vi "删除无效的文件路径.vi"(8 "error in (no error)":errorcluster, 10 "Enum":enum16{".xls", ".txt"}(ring), 11 "NewVal":string[](array[string])) -> (0 "error out":errorcluster, 2 "FilePathArray":path[](array[path]), 3 "NewVal 2":string[](array[string]))   [LabVIEW 2012]
doc: "从树形结构中选择的多个文件，有些是无效的文件路径（文件夹路径），需要删除。\n\nName:蒋松\nEmail:jiangsong@outlook.com"
panel:
  # "VI INPUTS"
  # "VI OUTPUTS"
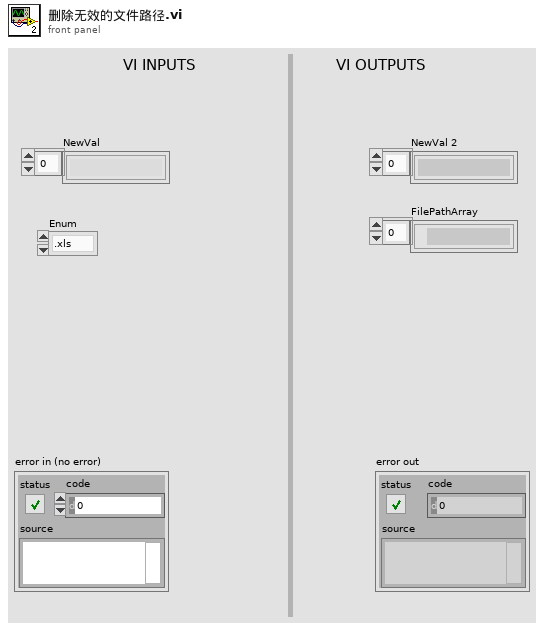
[diagram p1: front panel]
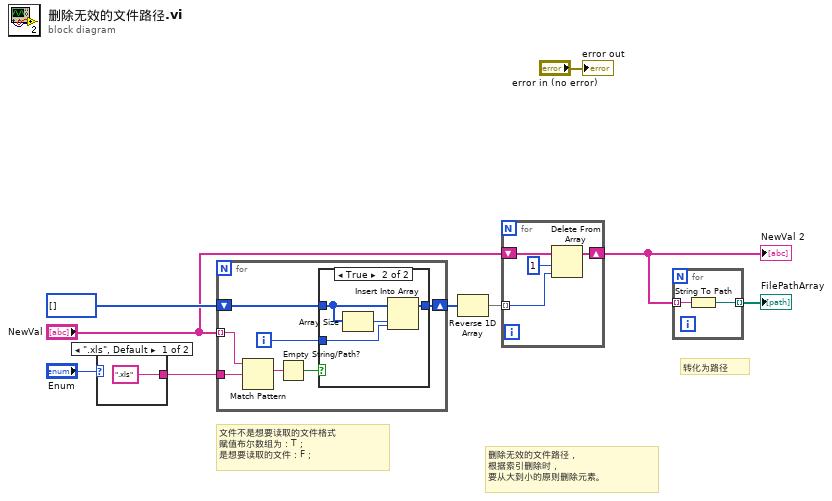
[diagram p0: block diagram]
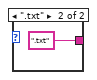
[diagram p2: hidden frame]
diagram:
  # "转化为路径"
  # "删除无效的文件路径，\n根据索引删除时，\n要从大到小的原则删除元素。"
  # "文件不是想要读取的文件格式\n赋值布尔数组为：T；\n是想要读取的文件：F；"
  n1 = case shown="\".xls\", Default" "Enum" {
    tunnel: [".xls" ".txt"] -> w5
    frame ".xls", Default {
    }
    frame ".txt" {
    }
  }
  n2 = for {
    tunnel: "NewVal" -> [w18] mode=indexing
    tunnel: w5 -> [w16]
    shift-right: [w12] -> w3
    shift-left: i32[] [] -> [w13]
    i -> [w14]
    n3 = Match Pattern(string=w18, regular expression=w16) -> (match substring=w17:string)  [unwired: 1 in, 3 out]
    n4 = Empty String/Path?(string/path=w17) -> (empty?=w15:bool)
    n5 = case shown="True" w15 {
      tunnel: w14 -> [_ w20]
      tunnel: w13 -> [w19 w22]
      tunnel: [w19 w23] -> w12
      frame False {
      }
      frame True {
        n6 = Array Size(array=w22) -> (size(s)=w21:i32)
        n7 = Insert Into Array(array=w22, index=w21, new element=w20) -> (w23:i32[])
      }
    }
  }
  n8 = Reverse 1D Array(array=w3) -> (reversed array=w1:i32[])
  n9 = for {
    shift-right: [w26] -> w8
    shift-left: "NewVal" -> [w27]
    tunnel: w1 -> [w24] mode=indexing
    n10 = Delete From Array(array=w27, length=1, index=w24) -> (array with subset deleted=w26:string[])  [unwired: 1 out]
  }
  "NewVal 2" <- w8
  n11 = for {
    tunnel: w8 -> [w29] mode=indexing
    tunnel: [w28] -> w7 mode=indexing
    n12 = String To Path(string=w29) -> (path=w28:path)
  }
  "FilePathArray" <- w7
  "error out" <- "error in (no error)"
